vi "Launcher.vi"   [LabVIEW 2020]
uses:
  First Actor.lvclass
  E:/Program Files (x86)/National Instruments/LabVIEW 2020/vi.lib/ActorFramework/Actor/Actor.lvclass
  First Actor Messages/PopUp Msg/PopUp Msg.lvclass/PopUp Msg.ctl
  <vilib>/ActorFramework/Message Enqueuer/Message Enqueuer.lvclass/Message Enqueuer.ctl
  <vilib>/ActorFramework/Message Enqueuer/Enqueue.vi
  First Actor Messages/PopUp Msg/PopUp Msg.lvclass
  E:/Program Files (x86)/National Instruments/LabVIEW 2020/vi.lib/ActorFramework/Message/Message.lvclass
  <vilib>/ActorFramework/Stop Msg/Stop Msg.lvclass
  <vilib>/ActorFramework/Message Priority Queue/Priority Enqueue.vi
  <vilib>/ActorFramework/Actor/Actor.lvclass
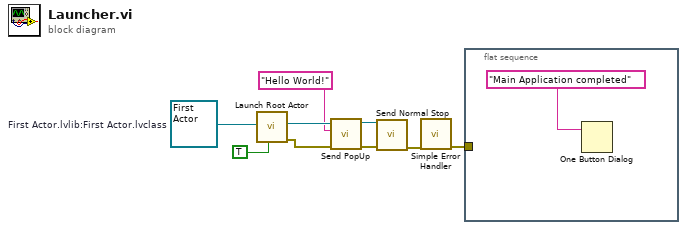
[diagram p0: block diagram]
diagram:
  w9 = refnum<class "First Actor.lvclass"> refnum  # First Actor.lvlib:First Actor.lvclass
  n1 = call <vilib>:"Launch Root Actor.vi"("Open Actor Core front panel? (F)"=TRUE, "Actor"=w9) -> ("error out"=w5:errorcluster, "Actor's Enqueuer"=w8:refnum<class "Message Enqueuer.lvclass">)  [unwired: 8 in]
  n2 = call "Send PopUp.vi"("error in (no error)"=w5, "String"="Hello World!", "Message Enqueuer"=w8) -> ("error out"=w4:errorcluster, "Message Enqueuer out"=w6:refnum<class "Message Enqueuer.lvclass">)  [unwired: 7 in]
  n3 = call <vilib>:"Send Normal Stop.vi"("error in (no error)"=w4, "Message Enqueuer"=w6) -> ("error out"=w3:errorcluster)  [unwired: 9 in]
  n4 = call <vilib>:"Simple Error Handler.vi"("error in (no error)"=w3) -> ("error out"=w1:errorcluster)  [unwired: 4 in, 4 out]
  n5 = flat-sequence {
    tunnel: w1 -> [_]
    frame #0 {
      n6 = One Button Dialog(message="Main Application completed") -> ()  [unwired: 1 in, 1 out]
    }
  }
